vi "DR200_control B_initialize.vi"(2 "B set (T)":dbl, 3 "Field Sweep Rate (T/min)":dbl min=-0.2 max=0.2, 4 "VISA Refnum in":refnum<visa-resource-name>) -> (1 "VISA Refnum out":refnum<visa-resource-name>)   [LabVIEW 2016]
uses:
  IPS120 - SubVIs/Typedefs/Set Activity - Enum.ctl
  IPS120 - SubVIs/IPS-120.lvlib
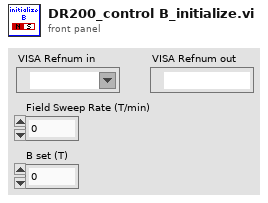
[diagram p1: front panel]
types:
  T1 = typedef "IPS-120.lvlib/Set Activity - Enum.ctl" = enum16{"Hold", "To Set Point", "To Zero", "Clamp"}
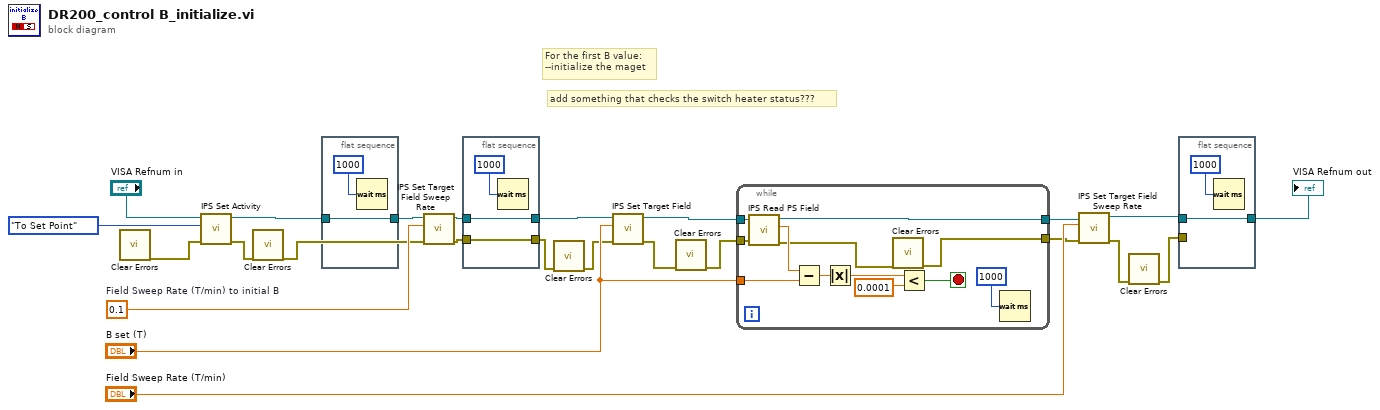
[diagram p0: block diagram]
diagram:
  w19 = 0.1  # Field Sweep Rate (T/min) to initial B
  # "add something that checks the switch heater status???"
  # "For the first B value:\n--initialize the maget"
  n1 = call <vilib>:"Clear Errors.vi"() -> ("error out"=w11:errorcluster)  [unwired: 6 in, 1 out]
  n2 = call "IPS Set Activity.vi"("Error In"=w11, "Set Activity"=Set_Activity_-_Enum."To Set Point", "VISA resource name"="VISA Refnum in") -> ("Error Out"=w10:errorcluster, "VISA resource name"=w13:refnum<visa-resource-name>)  [unwired: 2 in, 1 out]
  n3 = call <vilib>:"Clear Errors.vi"("error in (no error)"=w10) -> ("error out"=w9:errorcluster)  [unwired: 5 in, 1 out]
  n4 = flat-sequence {
    tunnel: w13 -> [w26]
    tunnel: [w26] -> w14
    frame #0 {
      n5 = Wait (ms)(milliseconds to wait=u32 1000) -> ()  [unwired: 1 out]
    }
  }
  n6 = call "IPS Set Target Field Sweep Rate.vi"("Error In"=w9, "Field Sweep Rate (T/min)"=w19, "VISA resource name"=w14) -> ("Error Out"=w12:errorcluster, "VISA resource name"=w21:refnum<visa-resource-name>)  [unwired: 2 in, 1 out]
  n7 = flat-sequence {
    tunnel: w21 -> [w29]
    tunnel: [w29] -> w20
    tunnel: w12 -> [w27]
    tunnel: [w27] -> w8
    frame #0 {
      n8 = Wait (ms)(milliseconds to wait=u32 1000) -> ()  [unwired: 1 out]
    }
  }
  n9 = call <vilib>:"Clear Errors.vi"("error in (no error)"=w8) -> ("error out"=w7:errorcluster)  [unwired: 5 in, 1 out]
  n10 = call "IPS Set Target Field.vi"("Error In"=w7, "Target Field (T)"="B set (T)", "VISA resource name"=w20) -> ("Error Out"=w5:errorcluster, "VISA resource name"=w24:refnum<visa-resource-name>)  [unwired: 2 in, 1 out]
  n11 = call <vilib>:"Clear Errors.vi"("error in (no error)"=w5) -> ("error out"=w4:errorcluster)  [unwired: 5 in, 1 out]
  n12 = while {
    tunnel: "B set (T)" -> [w33]
    tunnel: w24 -> [w35]
    tunnel: [w34] -> w17
    tunnel: w4 -> [w32]
    tunnel: [w30] -> w6
    stop <- w38 stop-if-true
    n13 = call "IPS Read PS Field.vi"("Error In"=w32, "VISA resource name"=w35) -> ("Error Out"=w31:errorcluster, "Field (T)"=w36:dbl, "VISA resource name"=w34:refnum<visa-resource-name>)  [unwired: 3 in]
    n14 = Subtract(x=w36, y=w33) -> (x-y=w40:dbl)
    n15 = Absolute Value(x=w40) -> (abs(x)=w39:dbl)
    n16 = call <vilib>:"Clear Errors.vi"("error in (no error)"=w31) -> ("error out"=w30:errorcluster)  [unwired: 5 in, 1 out]
    n17 = Less?(x=w39, y=0.0001) -> (x < y?=w38:bool)
    n18 = Wait (ms)(milliseconds to wait=u32 1000) -> ()  [unwired: 1 out]
  }
  n19 = call "IPS Set Target Field Sweep Rate.vi"("Error In"=w6, "Field Sweep Rate (T/min)"="Field Sweep Rate (T/min)", "VISA resource name"=w17) -> ("Error Out"=w3:errorcluster, "VISA resource name"=w16:refnum<visa-resource-name>)  [unwired: 2 in, 1 out]
  n20 = call <vilib>:"Clear Errors.vi"("error in (no error)"=w3) -> ("error out"=w2:errorcluster)  [unwired: 5 in, 1 out]
  n21 = flat-sequence {
    tunnel: w16 -> [w43]
    tunnel: [w43] -> w18
    tunnel: w2 -> [_]
    frame #0 {
      n22 = Wait (ms)(milliseconds to wait=u32 1000) -> ()  [unwired: 1 out]
    }
  }
  "VISA Refnum out" <- w18
